vi "System Status.vi"(7 "Box ID":u8=1, 8 "error in (no error)":errorcluster, 11 "CAN in":refnum<class "XNET_BS120x.lvclass">) -> (0 "error out":errorcluster, 2 "Status":T1, 3 "CAN out":refnum<class "XNET_BS120x.lvclass">)   [LabVIEW 2021, in "BS120x Driver.lvlib" / "XNET_BS120x.lvclass"]
uses:
  XNET_BS120x.lvclass
  TypeDefs/System Status.ctl
  BS120x.lvclass
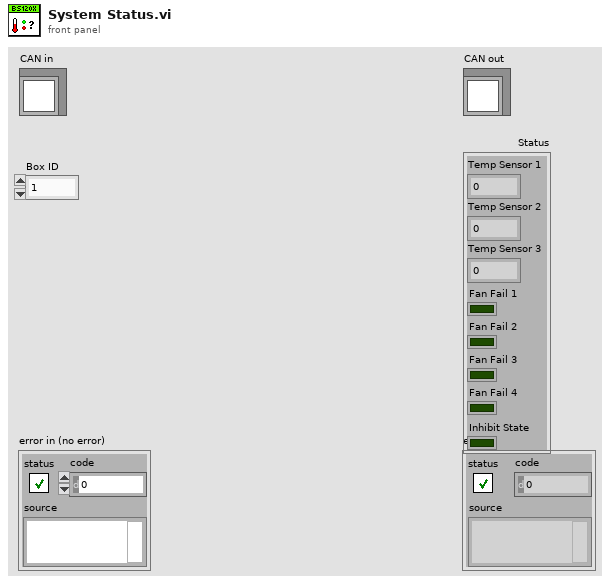
[diagram p1: front panel]
types:
  T1 = typedef "BS120x Driver.lvlib/BS120x.lvclass/System Status.ctl" = cluster{"Temp Sensor 1":dbl, "Temp Sensor 2":dbl, "Temp Sensor 3":dbl, "Fan Fail 1":bool, "Fan Fail 2":bool, "Fan Fail 3":bool, "Fan Fail 4":bool, "Inhibit State":bool}
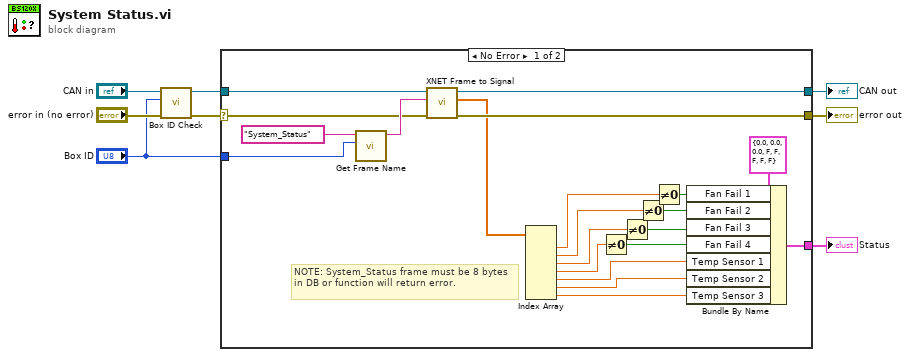
[diagram p0: block diagram]
diagram:
  n1 = call "Box ID Check.vi"("error in (no error)"="error in (no error)", "Box ID"="Box ID", "CAN in"="CAN in") -> ("error out"=w3:errorcluster, "CAN out"=w4:refnum<class "XNET_BS120x.lvclass">)  [unwired: 7 in]
  n2 = case shown="No Error" w3 {
    selector: w3 -> [w9 w30]
    tunnel: w4 -> [w29 w31]
    tunnel: [w28 w31] -> w7
    tunnel: [w27 w30] -> w6
    tunnel: [w13 _] -> w5
    tunnel: "Box ID" -> [w10 _]
    frame No Error {
      # "NOTE: System_Status frame must be 8 bytes in DB or function will return error."
      n3 = call "Get Frame Name.vi"("Box ID"=w10, "Frame Name"="System_Status" ("name")) -> ("Frame Name out"=w11:string)  [unwired: 9 in]
      n4 = call "XNET Frame to Signal.vi"("error in (no error)"=w9, "Frame"=w11, "CAN in"=w29) -> ("error out"=w27:errorcluster, "signal data"=w14:dbl[], "CAN out"=w28:refnum<class "XNET_BS120x.lvclass">)  [unwired: 6 in]
      n5 = Index Array(array=w14) -> (element #1=w21:dbl, element #2=w20:dbl, element #3=w19:dbl, element #4=w18:dbl, element #5=w17:dbl, element #6=w16:dbl, element #7=w22:dbl)  [unwired: 7 in]
      n6 = Not Equal To 0?(x=w18) -> (x != 0?=w24:bool)
      n7 = Not Equal To 0?(x=w19) -> (x != 0?=w23:bool)
      n8 = Not Equal To 0?(x=w20) -> (x != 0?=w25:bool)
      n9 = Not Equal To 0?(x=w21) -> (x != 0?=w26:bool)
      n10 = Bundle By Name(cluster=T1 {"Temp Sensor 1"=0.0, "Temp Sensor 2"=0.0, "Temp Sensor 3"=0.0, "Fan Fail 1"=FALSE, "Fan Fail 2"=FALSE, "Fan Fail 3"=FALSE, "Fan Fail 4"=FALSE, "Inhibit State"=FALSE} ("Status"), "Fan Fail 1"=w26, "Fan Fail 2"=w25, "Fan Fail 3"=w23, "Fan Fail 4"=w24, "Temp Sensor 1"=w17, "Temp Sensor 2"=w16, "Temp Sensor 3"=w22) -> (w13:T1)
    }
    frame Error {
    }
  }
  "error out" <- w6
  "CAN out" <- w7
  "Status" <- w5
